vi "server.vi"() -> ()   [LabVIEW 2024]
panel:
  in  "Historical Log Path":path
  out "Average Temperature (Last 5)":dbl
  in  "Password Input":string
  in  "Heater ON/OFF":bool
  out "System Status":enum16{"Automatic", "Manual"}(ring)
  out "Heater Status":T1(ring)
  out "Expected Ambient reading":dbl(slide) scale=0.0..100.0
  in  "Manual/Automatic switch":bool
  in  "Sample rate":dbl
  in  "Temperature setpoint control high":dbl
  in  "Temperature setpoint control low":dbl
  in  "Power ON/OFF":bool
  out "Historical temperature reading":dbl[](graph)
  out "Min temperature reading":dbl
  out "Max temperature reading":dbl
  out "Current temperature reading":dbl(slide) scale=0.0..100.0
  out "Heater ON/OFF":bool
  out "Power ON/OFF":bool
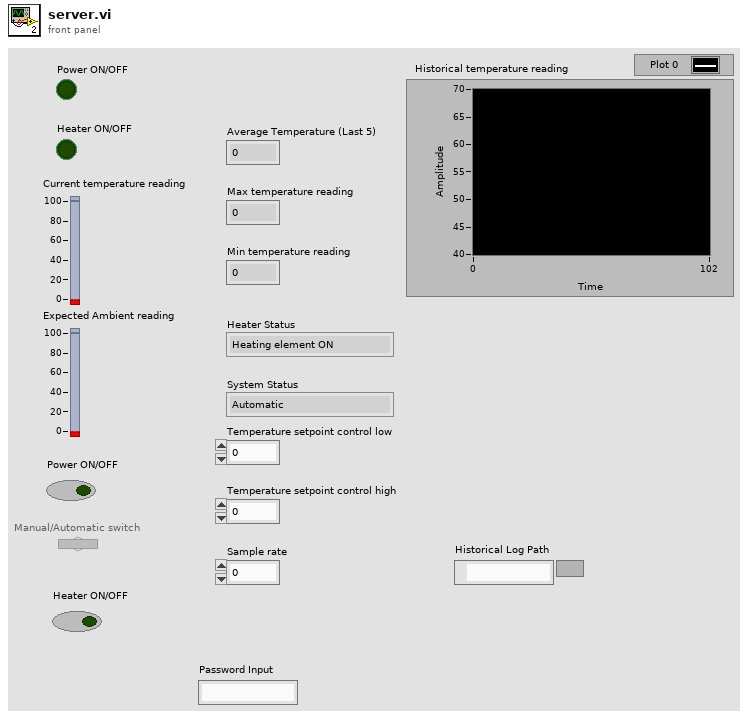
[diagram p1: front panel]
types:
  T1 = enum16{"Heating element ON", "Heating element OFF"}
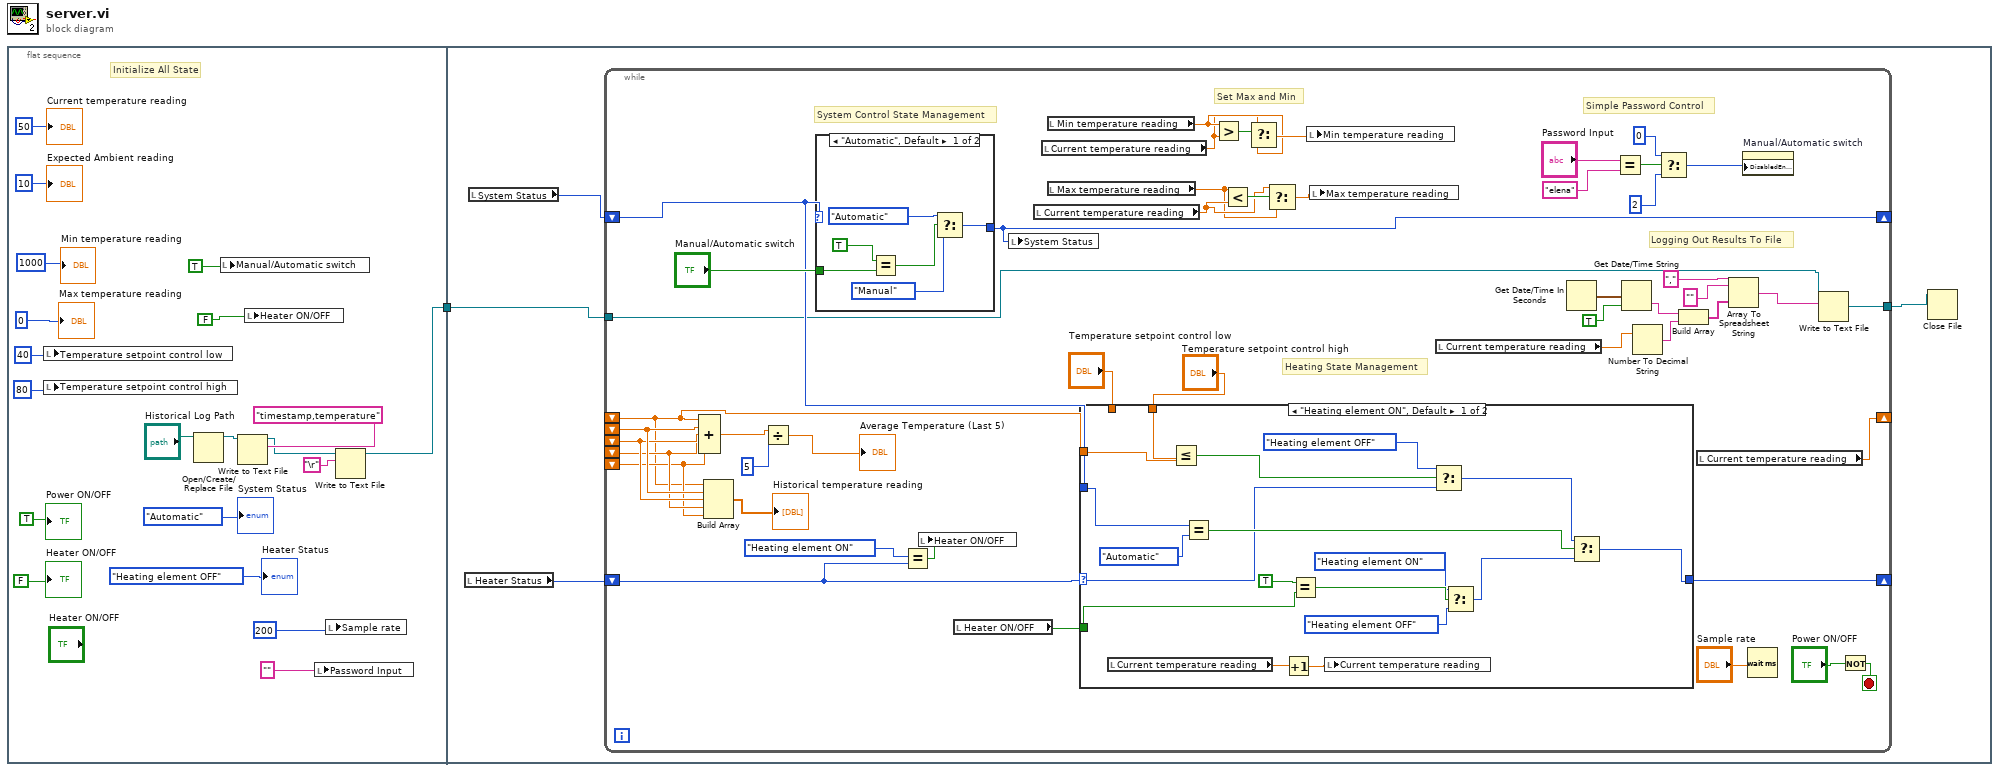
[diagram p0: block diagram]
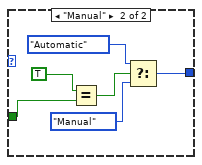
[diagram p2: hidden frame]
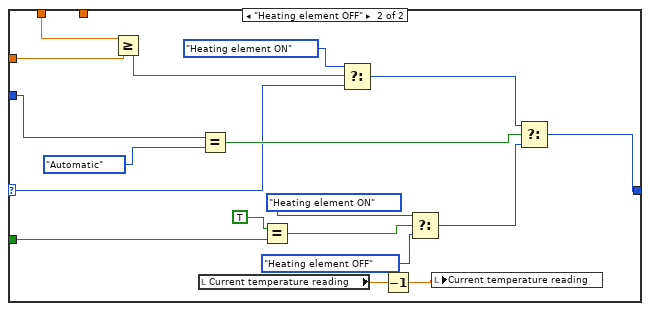
[diagram p3: hidden frame]
diagram:
  n1 = flat-sequence {
    tunnel: [w2] -> w1
    tunnel: w1 -> [w22]
    frame #0 {
      # "Initialize All State"
      n2 = local write "Temperature setpoint control low"(40) -> ()
      n3 = local write "Temperature setpoint control high"(80) -> ()
      n4 = Open/Create/Replace File(file path (use dialog)="Historical Log Path") -> (refnum out=w5:refnum<file>)  [unwired: 5 in, 2 out]
      n5 = local write "Manual/Automatic switch"(TRUE) -> ()
      n6 = Write to Text File(file (use dialog)=w5, text="timestamp,temperature") -> (refnum out=w4:refnum<file>)  [unwired: 2 in, 2 out]
      n7 = local write "Heater ON/OFF"(FALSE) -> ()
      n8 = local write "Password Input"("") -> ()
      n9 = local write "Sample rate"(200) -> ()
      n10 = Write to Text File(file (use dialog)=w4, text="\r") -> (refnum out=w2:refnum<file>)  [unwired: 2 in, 2 out]
      "Power ON/OFF" <- TRUE
      "Heater ON/OFF" <- FALSE
      "Current temperature reading" <- 50
      "Max temperature reading" <- 0
      "Min temperature reading" <- 1000
      "Expected Ambient reading" <- 10
      "System Status" <- enum16{"Automatic", "Manual"}."Automatic"
      "Heater Status" <- T1."Heating element OFF"
    }
    frame #1 {
      n11 = local read "Heater Status"() -> (w25:T1)
      n12 = local read "System Status"() -> (w24:enum16{"Automatic", "Manual"})
      n13 = while {
        shift-right: [w70] -> _
        shift-left: w25 -> [w56]
        shift-right: [w72] -> _
        shift-left: w24 -> [w59]
        shift-right: [w51] -> _
        shift-left: _ -> [w30]
        shift-left: _ -> [w50]
        shift-left: _ -> [w49]
        shift-left: _ -> [w48]
        shift-left: _ -> [w47]
        tunnel: [w41] -> w23
        tunnel: w22 -> [w31]
        stop <- w68 stop-if-true
        # "Set Max and Min"
        # "Logging Out Results To File"
        # "Simple Password Control"
        # "System Control State Management"
        # "Heating State Management"
        n14 = Compound Arithmetic op=ADD(w30, w50, w49, w48, w47) -> (w54:dbl)
        n15 = Build Array(w30, w50, w49, w48, w47) -> (→"Historical temperature reading":dbl[])
        n16 = Divide(x=w54, y=5) -> (x/y=→"Average Temperature (Last 5)":dbl)
        n17 = case shown="\"Automatic\", Default" w59 {
          tunnel: "Manual/Automatic switch" -> [w79 w81]
          tunnel: [w74 w80] -> w72
          frame "Automatic", Default {
            n18 = Equal?(x=TRUE, y=w79) -> (x = y?=w77:bool)
            n19 = Select(t=enum16{"Automatic", "Manual"}."Automatic", s=w77, f=enum16{"Automatic", "Manual"}."Manual") -> (s? t:f=w74:enum16{"Automatic", "Manual"})
          }
          frame "Manual" {
            n20 = Equal?(x=TRUE, y=w81) -> (x = y?=w84:bool)
            n21 = Select(t=enum16{"Automatic", "Manual"}."Automatic", s=w84, f=enum16{"Automatic", "Manual"}."Manual") -> (s? t:f=w80:enum16{"Automatic", "Manual"})
          }
        }
        n22 = Equal?(x=T1."Heating element ON", y=w56) -> (x = y?=w55:bool)
        n23 = local write "Heater ON/OFF"(w55) -> ()
        n24 = local read "Heater ON/OFF"() -> (w71:bool)
        n25 = local write "System Status"(w72) -> ()
        n26 = local read "Current temperature reading"() -> (w33:dbl)
        n27 = local read "Current temperature reading"() -> (w36:dbl)
        n28 = local read "Min temperature reading"() -> (w37:dbl)
        n29 = local read "Max temperature reading"() -> (w32:dbl)
        n30 = case shown="\"Heating element ON\", Default" w56 {
          selector: w56 -> [w87 w104]
          tunnel: [w88 w113] -> w70
          tunnel: w71 -> [w101 w117]
          tunnel: "Temperature setpoint control high" -> [w96 _]
          tunnel: "Temperature setpoint control low" -> [_ w106]
          tunnel: w30 -> [w95 w105]
          tunnel: w59 -> [w91 w110]
          frame "Heating element ON", Default {
            n31 = local read "Current temperature reading"() -> (w98:dbl)
            n32 = Less Or Equal?(x=w96, y=w95) -> (x <= y?=w86:bool)
            n33 = Equal?(x=w91, y=enum16{"Automatic", "Manual"}."Automatic") -> (x = y?=w89:bool)
            n34 = Increment(x=w98) -> (x+1=w97:dbl)
            n35 = Equal?(x=TRUE, y=w101) -> (x = y?=w102:bool)
            n36 = local write "Current temperature reading"(w97) -> ()
            n37 = Select(t=T1."Heating element OFF", s=w86, f=w87) -> (s? t:f=w93:T1)
            n38 = Select(t=T1."Heating element ON", s=w102, f=T1."Heating element OFF") -> (s? t:f=w92:T1)
            n39 = Select(t=w93, s=w89, f=w92) -> (s? t:f=w88:T1)
          }
          frame "Heating element OFF" {
            n40 = Greater Or Equal?(x=w106, y=w105) -> (x >= y?=w107:bool)
            n41 = local read "Current temperature reading"() -> (w116:dbl)
            n42 = Equal?(x=w110, y=enum16{"Automatic", "Manual"}."Automatic") -> (x = y?=w108:bool)
            n43 = Equal?(x=TRUE, y=w117) -> (x = y?=w120:bool)
            n44 = Select(t=T1."Heating element ON", s=w107, f=w104) -> (s? t:f=w111:T1)
            n45 = Decrement(x=w116) -> (x-1=w115:dbl)
            n46 = Select(t=T1."Heating element ON", s=w120, f=T1."Heating element OFF") -> (s? t:f=w112:T1)
            n47 = local write "Current temperature reading"(w115) -> ()
            n48 = Select(t=w111, s=w108, f=w112) -> (s? t:f=w113:T1)
          }
        }
        n49 = Greater?(x=w37, y=w36) -> (0:w39:bool)
        n50 = Less?(x=w32, y=w33) -> (x < y?=w35:bool)
        n51 = Select(t=w36, s=w39, f=w37) -> (s? t:f=w38:dbl)
        n52 = Select(t=w33, s=w35, f=w32) -> (s? t:f=w34:dbl)
        n53 = local write "Min temperature reading"(w38) -> ()
        n54 = local write "Max temperature reading"(w34) -> ()
        n55 = local read "Current temperature reading"() -> (w26:dbl)
        n56 = Get Date/Time In Seconds() -> (seconds since 1Jan1904=w45:timestamp)
        n57 = Equal?(x="Password Input", y="elena") -> (x = y?=w64:bool)
        n58 = Get Date/Time String(seconds (now)=w45, want seconds? (F)=TRUE) -> (time string=w44:string)  [unwired: 1 in, 1 out]
        n59 = Number To Decimal String(number=w26) -> (decimal integer string=w40:string)  [unwired: 1 in]
        n60 = Select(t=0, s=w64, f=2) -> (s? t:f=w67:i32)
        n61 = Build Array(w44, w40) -> (w43:string[])
        n62 = local read "Current temperature reading"() -> (w51:dbl)
        n63 = Array To Spreadsheet String(delimiter (Tab)=",", array=w43, 3:"") -> (spreadsheet string=w42:string)
        n64 = property on="Manual/Automatic switch" class="Bool (strict)"("DisabledEnum"=w67) -> ()  [unwired: 2 in, 2 out]
        n65 = Wait (ms)(milliseconds to wait="Sample rate") -> ()  [unwired: 1 out]
        n66 = Write to Text File(file (use dialog)=w31, text=w42) -> (refnum out=w41:refnum<file>)  [unwired: 2 in, 2 out]
        n67 = Not(x="Power ON/OFF") -> (.not. x?=w68:bool)
      }
      n68 = Close File(refnum=w23) -> ()  [unwired: 1 in, 2 out]
    }
  }
